vi "Example Drag and  Drop.vi"() -> ()   [LabVIEW 2021]
uses:
  <vilib>/Utility/miscctls.llb/LVPoint32TypeDef.ctl
  <vilib>/Utility/miscctls.llb/LVRectTypeDef.ctl
panel:
  out "old Front Panel Window:Panel Bounds":T1
  out "error out":errorcluster
  out "current time":timestamp
  out "Coords 2":T2
  out "drag target":picture
  in  "stop":bool
  out "Tank":picture
  # "Question: how do we make the live VI, such as the feed module graphic\nsized right for the picture that is loaded?\n\nProbably should standarize each module size. Then the  flow sheet\ndrawings will all just match the size and we don't have to worry about\nscale."
  # "Tasks\n1. Load graphic\n2. Drag and drop onto picture control\n3. Picture control draws hot spot\n4. If drag and drop on picture control, then resize and redraw the nearest hotspot\n5. When operator turns \"ON\" the system, then the hotspots are replaced with actual VIs."
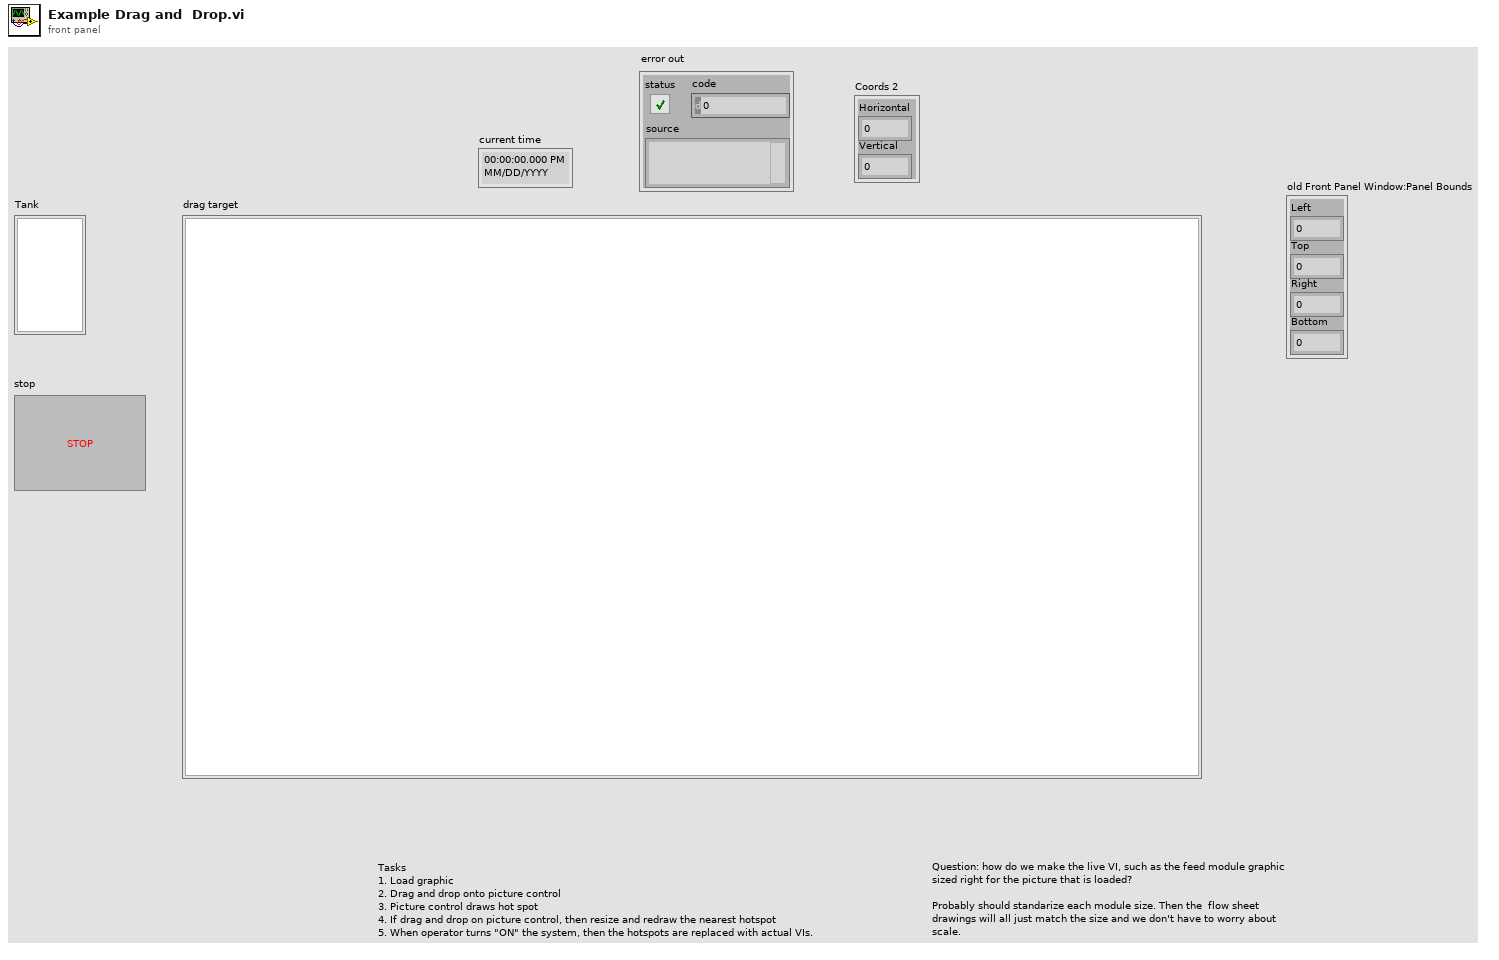
[diagram p1: front panel]
types:
  T1 = typedef "LVRectTypeDef.ctl" = cluster{"Left":i16, "Top":i16, "Right":i16, "Bottom":i16}
  T2 = typedef "LVPoint32TypeDef.ctl" = cluster{"Horizontal":i32, "Vertical":i32}
  T3 = typedef "imagedata.ctl" = cluster{"image type":i32, "image depth":i32, "image":u8[], "mask":u8[], "colors":u32[], "Rectangle":cluster{"left":i16, "top":i16, "right":i16, "bottom":i16}}
  T4 = typedef "LVPointTypeDef.ctl" = cluster{"Horizontal":i16, "Vertical":i16}
  T5 = enum32{"Invalid", "Standard", "Closed", "Hidden", "Minimized", "Maximized"}
  T6 = cluster{"data name":string, "drag data":variant}[]
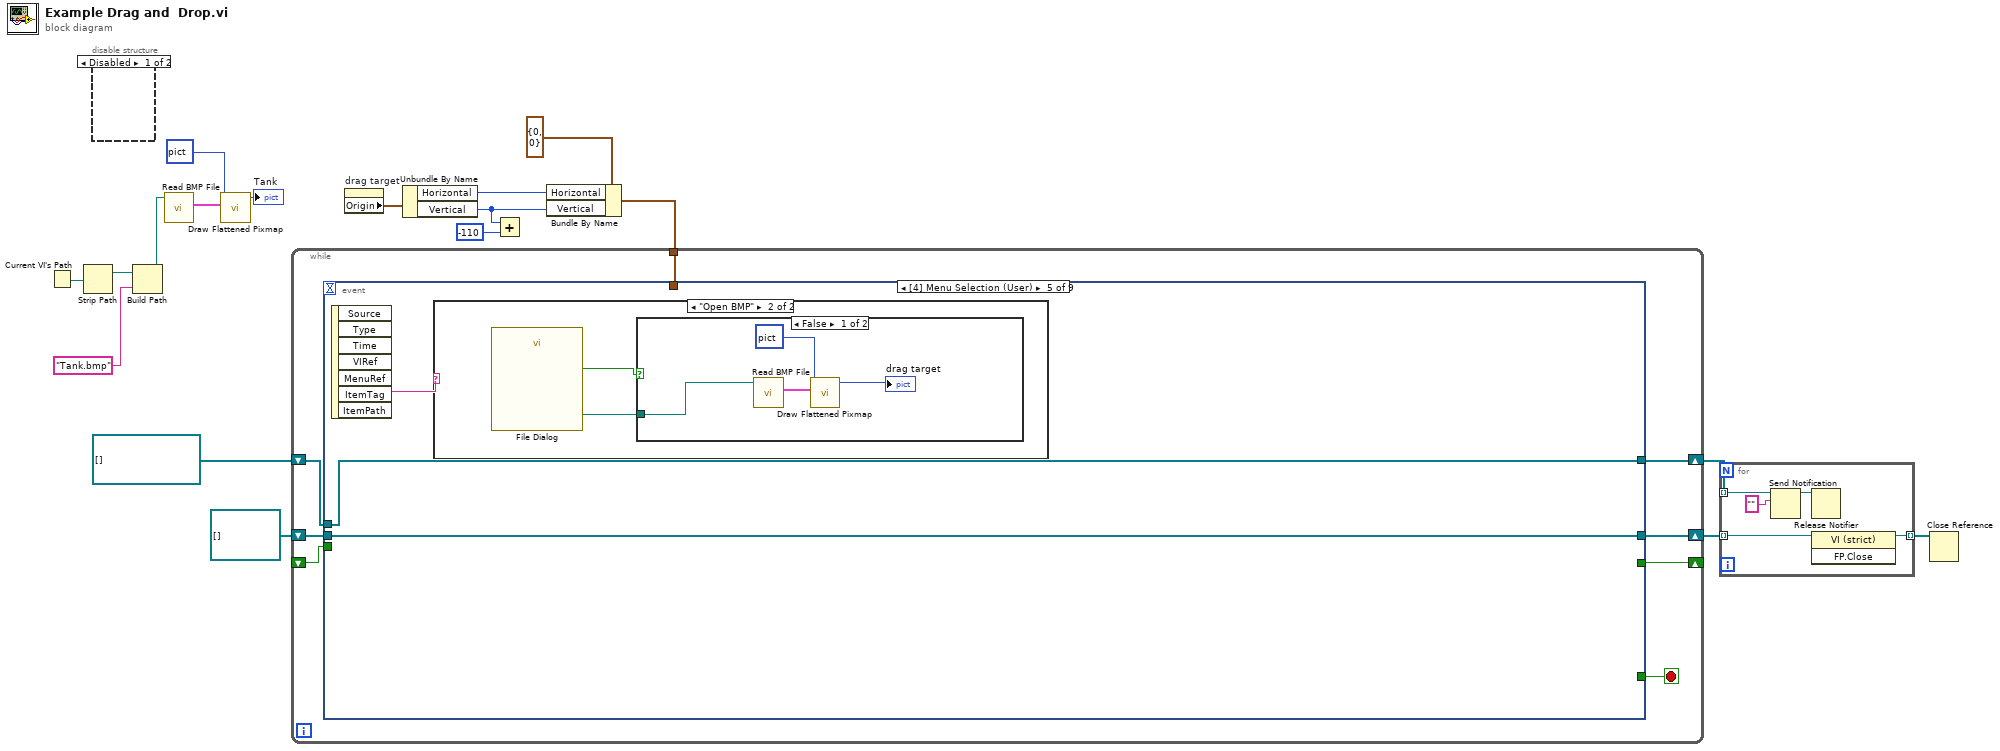
[diagram p0: block diagram]
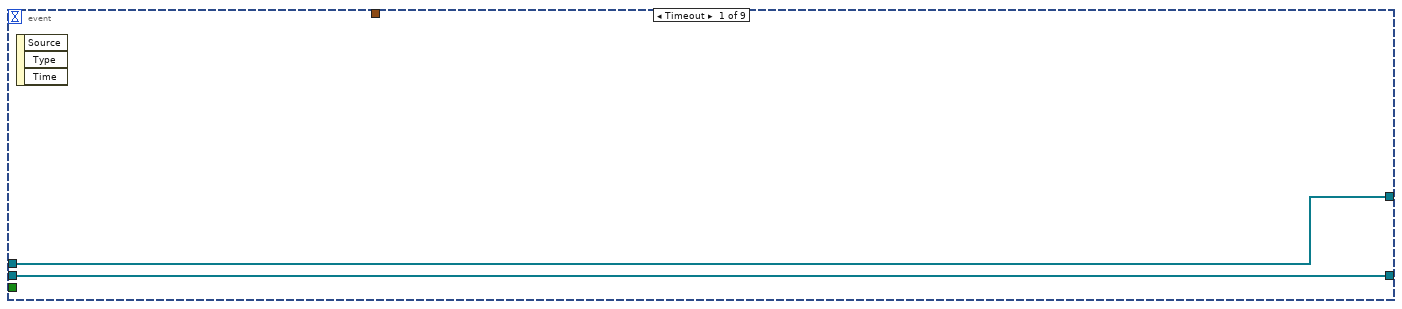
[diagram p3: hidden frame]
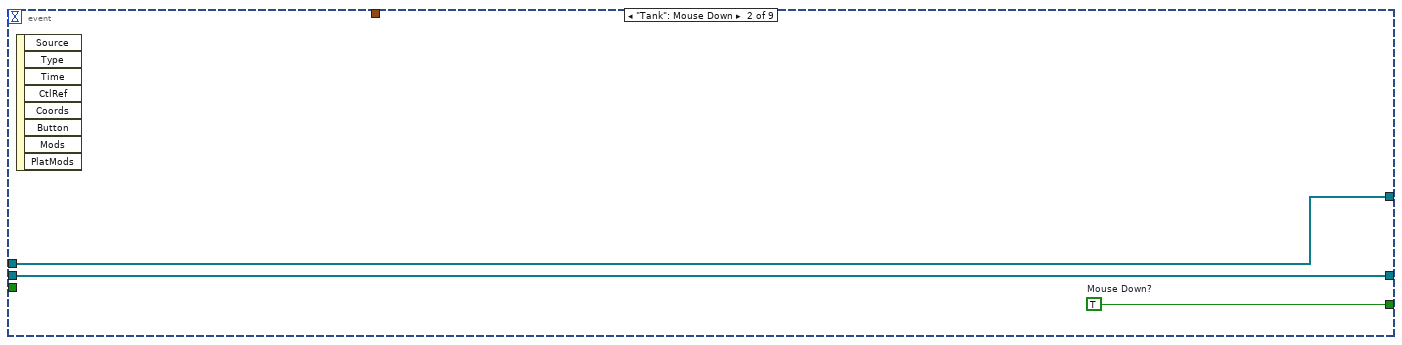
[diagram p4: hidden frame]
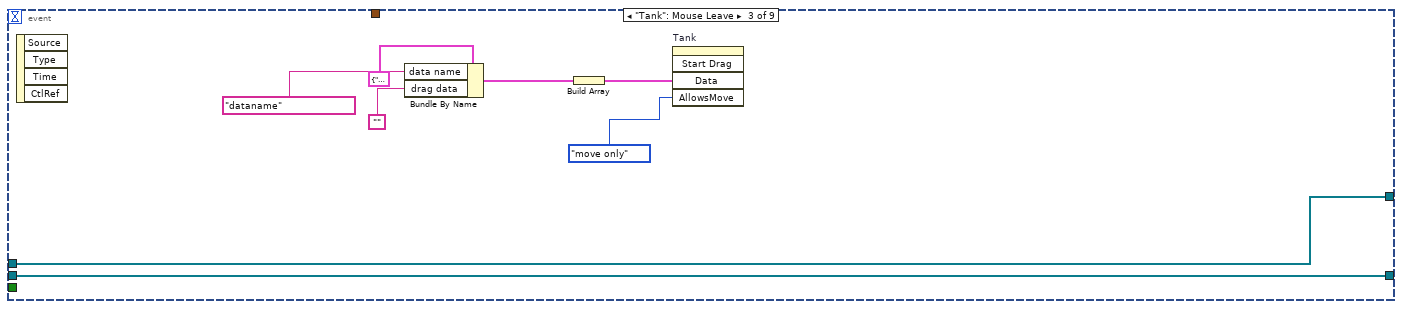
[diagram p5: hidden frame]
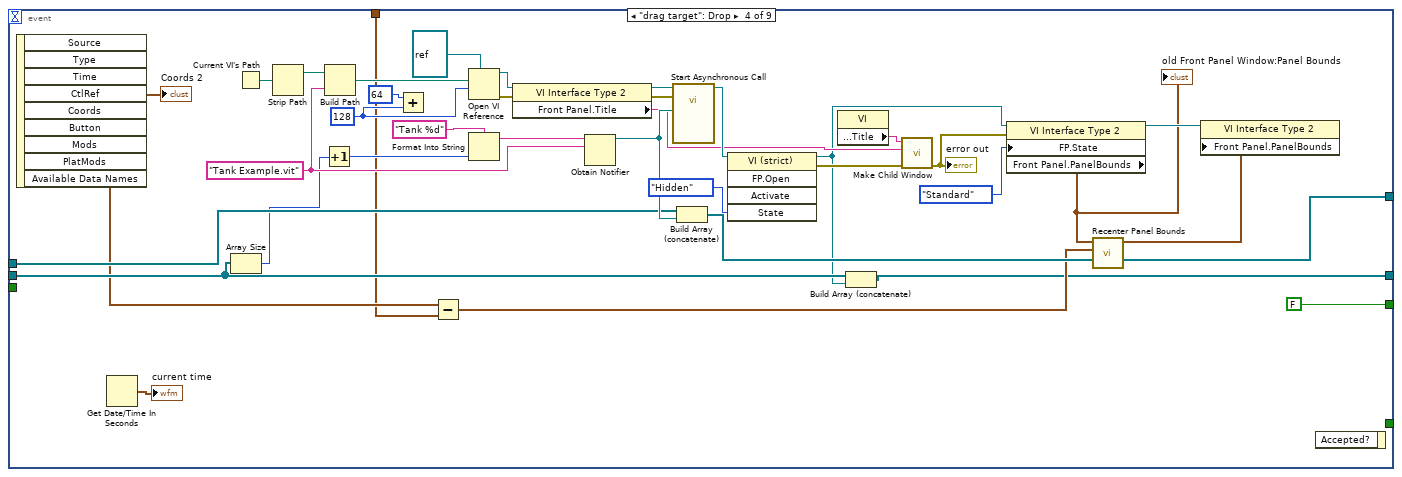
[diagram p6: hidden frame]
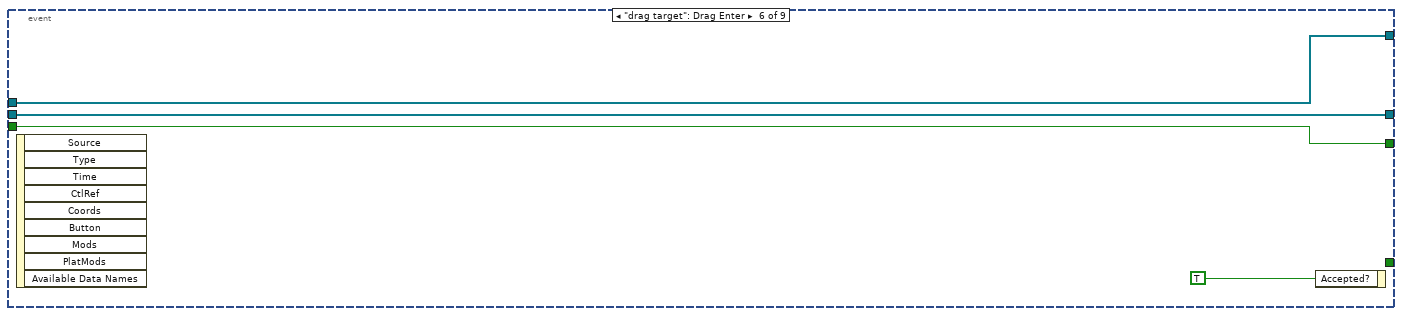
[diagram p9: hidden frame]
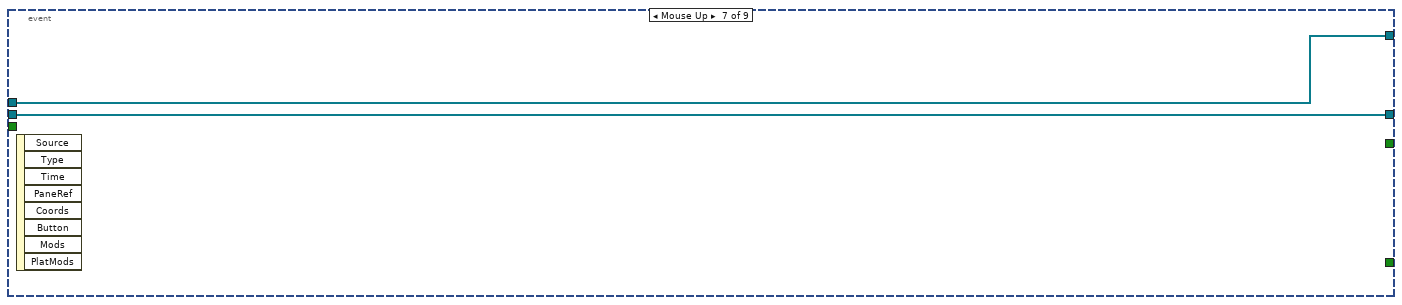
[diagram p10: hidden frame]
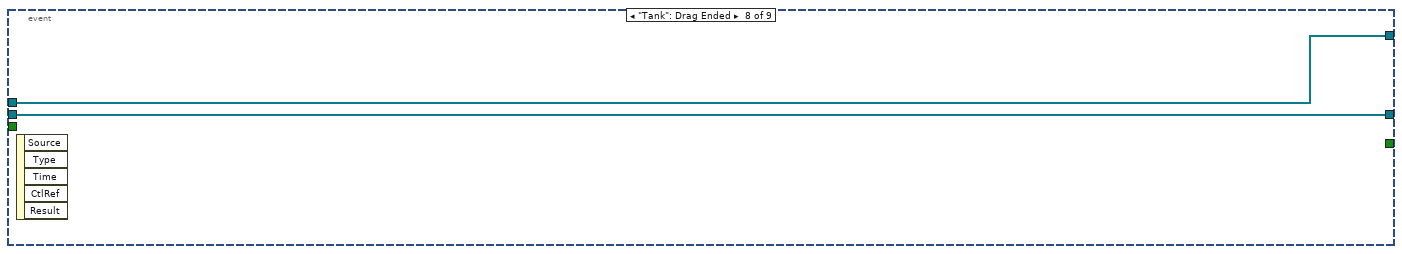
[diagram p11: hidden frame]
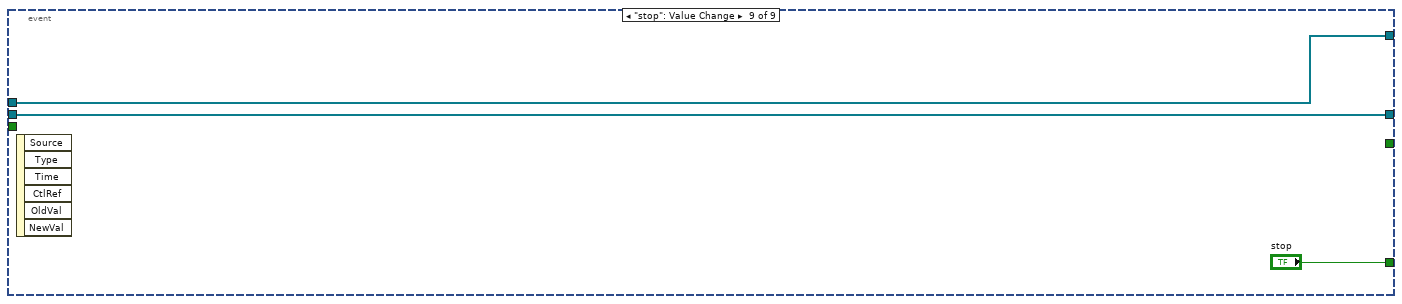
[diagram p12: hidden frame]
diagram:
  n1 = Current VI's Path() -> (path=w6:path)
  n2 = Strip Path(path=w6) -> (stripped path=w7:path)  [unwired: 1 out]
  n3 = disable-structure shown="Disabled" {
    frame Disabled {
    }
    frame Enabled {
    }
  }
  n4 = Build Path(base path=w7, name or relative path="Tank.bmp") -> (appended path=w2:path)
  n5 = call <vilib>:"Read BMP File.vi"("path to BMP file"=w2) -> ("image data"=w3:T3)  [unwired: 8 in, 2 out]
  n6 = call <vilib>:"Draw Flattened Pixmap.vi"("image data"=w3, "picture"=picture data[5B]) -> ("new picture"=→"Tank":picture)  [unwired: 7 in]
  n7 = property on="drag target" class="Pict"() -> ("Origin"=w10:T4)  [unwired: 2 in, 2 out]
  n8 = Unbundle By Name(w10) -> ("Horizontal"=w12:i16, "Vertical"=w8:i16)
  n9 = Add(x=w8, y=i16 -110) -> ()  [unwired: 1 out]
  n10 = Bundle By Name(cluster=T2 {"Horizontal"=0, "Vertical"=0} ("Coords 2"), "Horizontal"=w12, "Vertical"=w8) -> (w11:T2)
  n11 = while {
    shift-right: [w25] -> _
    shift-left: _ -> [w24]
    shift-right: [w23] -> w16
    shift-left: refnum<vi>[] [] -> [w22]
    shift-right: [w21] -> w14
    shift-left: refnum<notifier>[] [] -> [w20]
    tunnel: w11 -> [w19]
    stop <- w26 stop-if-true
    n12 = event shown="[4] Menu Selection (User)" {
      selector: _ -> [_ _ _ _ _ _ _ _ _]
      dyn-events: _ -> [_ _ _ _ _ _ _ _ _]
      timeout: _ -> [_ _ _ _ _ _ _ _ _]
      tunnel: [_ _ _ _ _ _ _ _ "stop"] -> w26
      tunnel: [_ w31 _ FALSE ("Mouse Down?") _ w87 _ _ _] -> w25
      tunnel: w24 -> [_ _ _ _ _ w87 _ _ _]
      tunnel: [w28 w30 w33 w40 w78 w86 w90 w92 w94] -> w23
      tunnel: w22 -> [w28 w30 w33 w63 w78 w86 w90 w92 w94]
      tunnel: [w27 w29 w32 w65 w77 w85 w89 w91 w93] -> w21
      tunnel: w20 -> [w27 w29 w32 w64 w77 w85 w89 w91 w93]
      tunnel: w19 -> [_ _ _ w45 _ _ _ _ _]
      event Timeout {
        n13 = event-data() -> ()  [unwired: 1 in, 3 out]
      }
      event "Tank": Mouse Down {
        w31 = TRUE  # Mouse Down?
        n14 = event-data() -> ()  [unwired: 1 in, 8 out]
      }
      event "Tank": Mouse Leave {
        n15 = event-data() -> ()  [unwired: 1 in, 4 out]
        n16 = Bundle By Name(cluster=cluster{"data name":string, "drag data":variant} {"data name"="", "drag data"=variant}, "data name"="dataname", "drag data"="") -> (w35:cluster{"data name":string, "drag data":variant})
        n17 = Build Array(w35) -> (w38:T6)
        n18 = invoke on="Tank" class="Pict" method="Start Drag"("Data"=w38, "AllowsMove"=enum32{"copy or move", "copy only", "move only"}."move only" ("Drag Mode")) -> ()  [unwired: 3 in, 5 out]
      }
      event "drag target": Drop {
        w68 = 128 ("options")
        w69 = "Tank Example.vit" ("name or relative path")
        n19 = event-data() -> ("Coords"=w46:T2)  [unwired: 1 in, 8 out]
        "Coords 2" <- w46
        n20 = Get Date/Time In Seconds() -> (seconds since 1Jan1904=→"current time":timestamp)
        n21 = Array Size(array=w63) -> (size(s)=w62:i32)
        n22 = Current VI's Path() -> (path=w72:path)
        n23 = Strip Path(path=w72) -> (stripped path=w73:path)  [unwired: 1 out]
        n24 = Increment(x=w62) -> (x+1=w60:i32)
        n25 = Build Path(base path=w73, name or relative path=w69) -> (appended path=w74:path)
        n26 = Add(x=64 ("options"), y=w68) -> ()  [unwired: 1 out]
        n27 = Subtract(x=w46, y=w45) -> (x-y=w42:T2)
        n28 = Open VI Reference(type specifier VI Refnum (for type only)=refnum<vi> refnum, vi path=w74, options=w68) -> (vi reference=w55:refnum<vi>, error out=w53:errorcluster)  [unwired: 3 in]
        n29 = Format Into String(format string="Tank %d", w60) -> (resulting string=w59:string)  [unwired: 2 in, 1 out]
        n30 = property class="VI Interface Type 2"(reference=w55, error in=w53) -> (reference out=w54:refnum<vi>, error out=w52:errorcluster, "Front Panel.Title"=w51:string)
        n31 = Obtain Notifier(name (unnamed)=w59, notification data type=w69) -> (notifier out=w66:refnum<notifier>)  [unwired: 2 in, 2 out]
        n32 = call-by-ref "Start Asynchronous Call"(reference=w54, error in=w52, "notifier"=w66) -> (reference out=w67:refnum<vi>)  [unwired: 11 in, 1 out]
        n33 = Build Array (concatenate)(w64, w66) -> (w65:refnum<notifier>[])
        n34 = invoke class="VI (strict)" method="FP.Open"(reference=w67, "State"=T5."Hidden") -> (reference out=w49:refnum<vi>, error out=w56:errorcluster)  [unwired: 3 in, 3 out]
        n35 = property class="VI"() -> ("Front Panel.Title"=w57:string)  [unwired: 2 in, 2 out]
        n36 = Build Array (concatenate)(w63, w49) -> (w40:refnum<vi>[])
        n37 = call "Make Child Window.vi"("error in (no error)"=w56, "Name of Child Panel"=w51, "Name of Parent Panel"=w57) -> ("error out"=w47:errorcluster)  [unwired: 4 in]
        "error out" <- w47
        n38 = property class="VI Interface Type 2"(reference=w49, error in=w47, "FP.State"=T5."Standard" ("Front Panel Window:State")) -> (reference out=w44:refnum<vi>, "Front Panel.PanelBounds"=w41:T1)  [unwired: 1 out]
        "old Front Panel Window:Panel Bounds" <- w41
        n39 = call "Recenter Panel Bounds.vi"("New Center Coords"=w42, "Front Panel Window:Panel Bounds in"=w41) -> ("Front Panel Window:Panel Bounds out"=w43:T1)  [unwired: 9 in]
        n40 = property class="VI Interface Type 2"(reference=w44, "Front Panel.PanelBounds"=w43) -> ()  [unwired: 1 in, 2 out]
        n41 = event-data() -> ()  [unwired: 2 in, 1 out]
      }
      event Menu Selection (User) {
        n42 = event-data() -> ("ItemTag"=w76:string)  [unwired: 1 in, 6 out]
        n43 = case shown="\"Open BMP\"" w76 {
          frame "False", Default {
          }
          frame "Open BMP" {
            n44 = call "File Dialog"() -> ("selected path"=w79:path, "cancelled"=w80:bool)  [unwired: 12 in, 2 out]
            n45 = case shown="False" w80 {
              tunnel: w79 -> [w84 _]
              frame False {
                n46 = call <vilib>:"Read BMP File.vi"("path to BMP file"=w84) -> ("image data"=w82:T3)  [unwired: 8 in, 2 out]
                n47 = call <vilib>:"Draw Flattened Pixmap.vi"("image data"=w82, "picture"=picture data[5B]) -> ("new picture"=→"drag target":picture)  [unwired: 7 in]
              }
              frame True {
              }
            }
          }
        }
      }
      event "drag target": Drag Enter {
        n48 = event-data() -> ()  [unwired: 1 in, 9 out]
        n49 = event-data("Accepted?"=TRUE) -> ()  [unwired: 1 in, 1 out]
      }
      event Mouse Up {
        n50 = event-data() -> ()  [unwired: 1 in, 8 out]
      }
      event "Tank": Drag Ended {
        n51 = event-data() -> ()  [unwired: 1 in, 5 out]
      }
      event "stop": Value Change {
        n52 = event-data() -> ()  [unwired: 1 in, 6 out]
      }
    }
  }
  n53 = for {
    tunnel: [w97] -> w17 mode=indexing
    tunnel: w16 -> [w96] mode=indexing
    tunnel: w14 -> [w99] mode=indexing
    n54 = Send Notification(notification="", notifier=w99) -> (notifier out=w98:refnum<notifier>)  [unwired: 1 in, 1 out]
    n55 = Release Notifier(notifier=w98) -> ()  [unwired: 2 in, 3 out]
    n56 = invoke class="VI (strict)" method="FP.Close"(reference=w96) -> (reference out=w97:refnum<vi>)  [unwired: 2 in, 2 out]
  }
  n57 = Close Reference(reference=w17) -> ()  [unwired: 1 in, 1 out]
